vi "OD.vi"() -> ()   [LabVIEW 2012]
uses:
  <vilib>/Instr/_visa.llb/VISA Find Search Mode.ctl
  <vilib>/Utility/file.llb/Read From Spreadsheet File (string).vi
  <vilib>/Utility/file.llb/Write To Spreadsheet File (string).vi
  <vilib>/Utility/file.llb/Write To Spreadsheet File (DBL).vi
  <userlib>/SPECcon/SPECcon.lvlib
panel:
  out "Dark 2":dbl[](array[numeric])
  in  "DarkBefore":bool
  in  "Interval in minutes":dbl
  out "Absorbance [AU] vs. Wavelength [nm]":cluster{dbl[], dbl[]}[](graph)
  in  "Reset the graph for\nnext run":bool
  out "Dark":dbl[](array[numeric])
  out "Reference":dbl[](array[numeric])
  out "Connected?":bool
  out "Identified?":bool
  in  "to":i32=1050
  in  "from":i32=350
  in  "Run Python Script\non 'log_OD.txt'":bool
  in  "Automatic\nMeasurement":bool
  out "Samples Raw Data":dbl[][][](array[numeric])
  out "Command sent":string
  out "Raw Data":string
  in  "Average":i32=10
  in  "Integration Time":i32=100
  out "Number of bytes read":i32
  out "info out":string
  out "info return":i32
  in  "Connect to this port?":bool caption="Connect to this port"
  in  "index":i32
  out "Port":string caption="element"
  out "firmware out":string
  # "Connection"
  # "Data Acquisition"
  # "Measurement Settings"
  # "Wavelength Range (nm)"
  # "-"
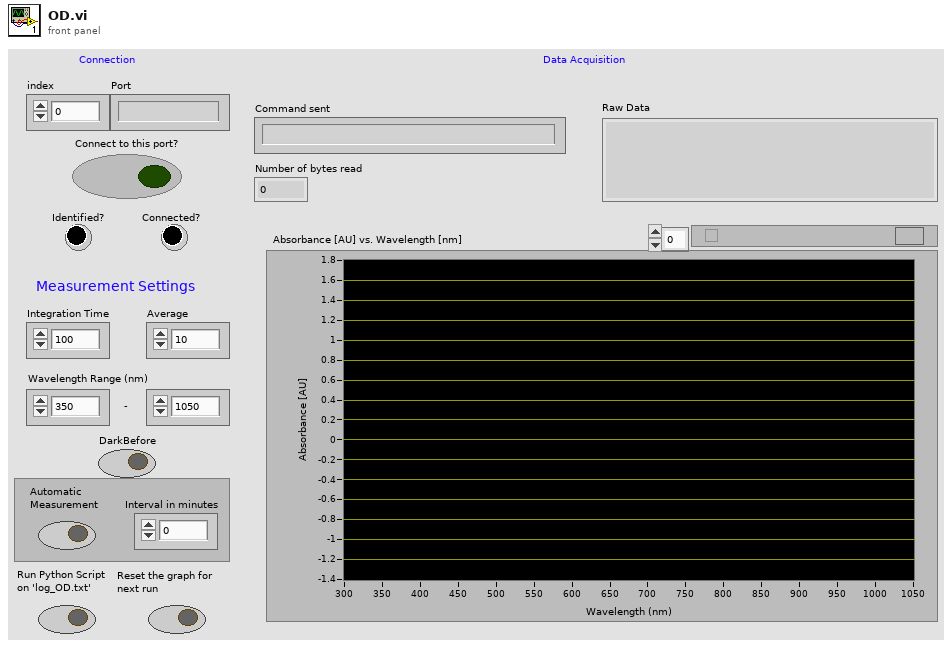
[diagram p1: front panel]
types:
  T1 = typedef "VISA Find Search Mode.ctl" = u32
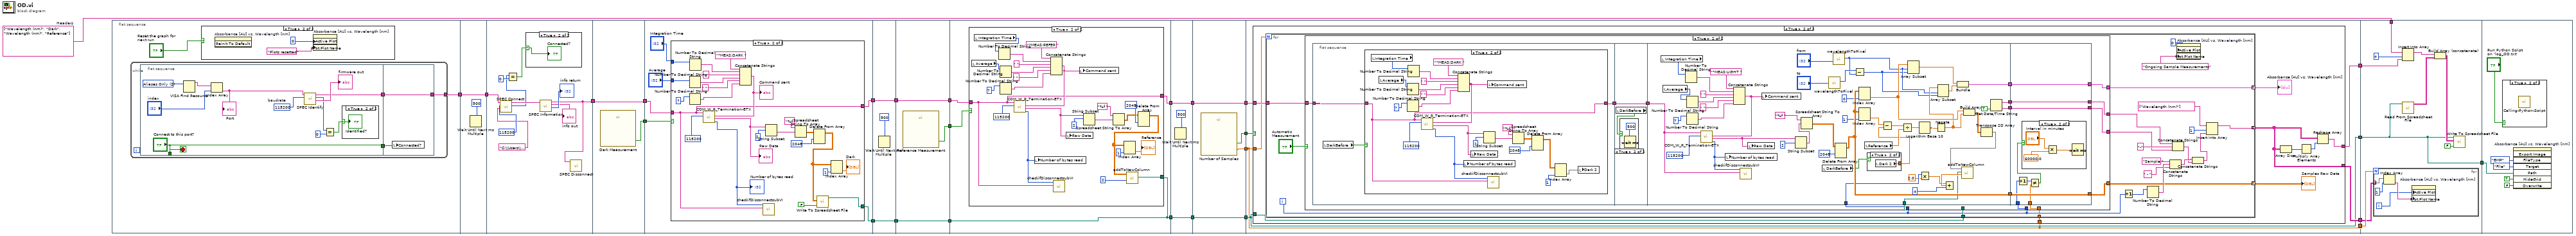
[diagram p0: block diagram]
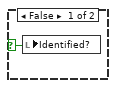
[diagram p3: hidden frame]
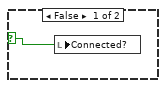
[diagram p4: hidden frame]
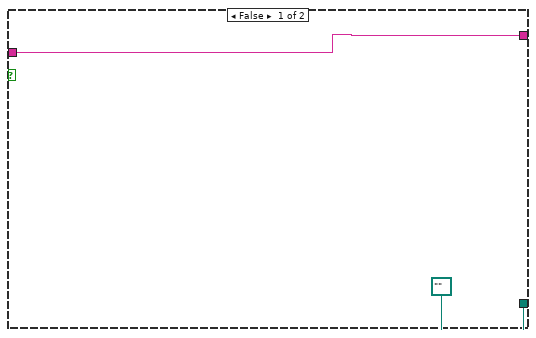
[diagram p5: hidden frame]
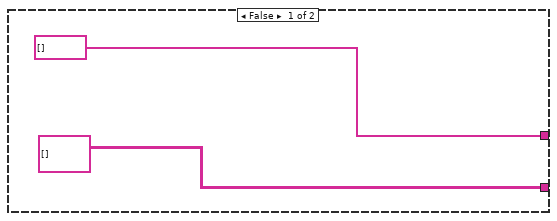
[diagram p7: hidden frame]
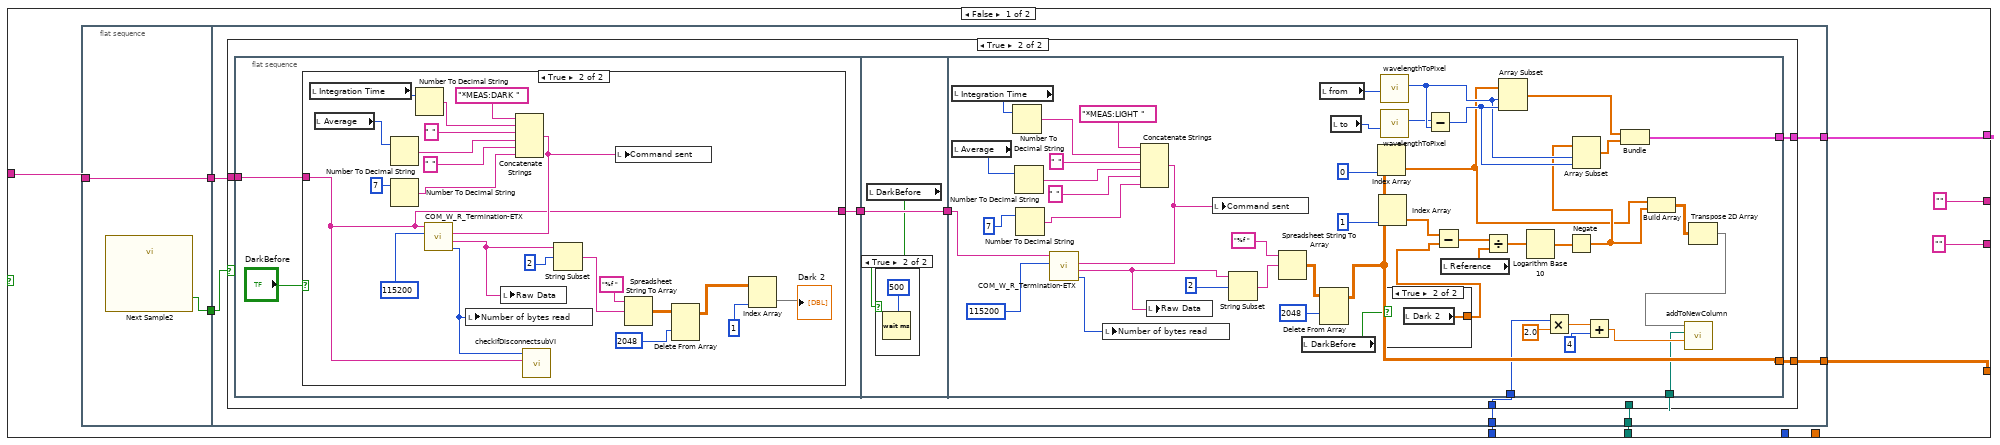
[diagram p8: hidden frame]
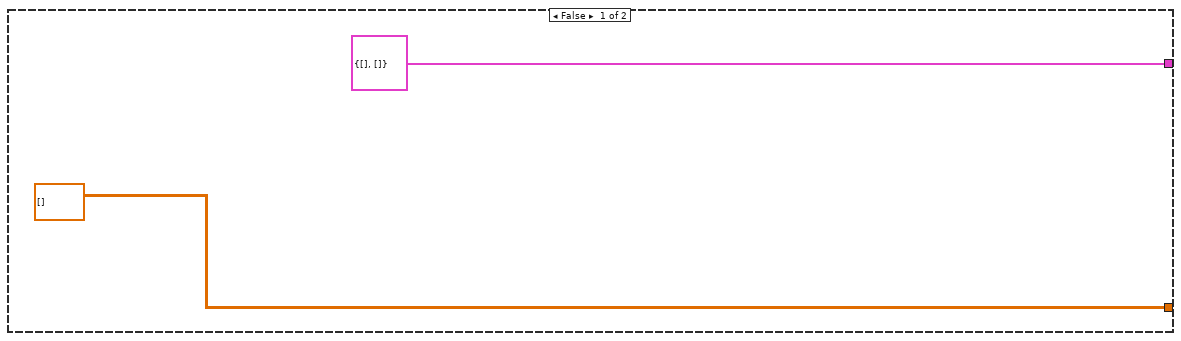
[diagram p9: hidden frame]
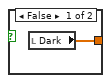
[diagram p12: hidden frame]
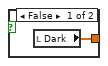
[diagram p15: hidden frame]
diagram:
  w5 = string[] ["Wavelength (nm)", "Dark", "Wavelength (nm)", "Reference"]  # Headers
  n1 = flat-sequence {
    tunnel: [w28] -> w26
    tunnel: w26 -> [w50]
    tunnel: [w50] -> w25
    tunnel: w25 -> [w58]
    tunnel: [w55] -> w16
    tunnel: [w65] -> w24
    tunnel: w16 -> [w65]
    tunnel: [w64] -> w15
    tunnel: w24 -> [w70]
    tunnel: w15 -> [w71]
    tunnel: [w67] -> w13
    tunnel: [w66] -> w7
    tunnel: [w99] -> w22
    tunnel: w13 -> [w99]
    tunnel: [w98] -> w8
    tunnel: w7 -> [w98]
    tunnel: [w103] -> w23
    tunnel: w22 -> [w103]
    tunnel: [w102] -> w21
    tunnel: [w101] -> w9
    tunnel: w8 -> [w101]
    tunnel: w23 -> [w107]
    tunnel: w21 -> [w106]
    tunnel: [w105] -> w14
    tunnel: [w104] -> w10
    tunnel: w9 -> [w104]
    tunnel: [w134] -> w17
    tunnel: w14 -> [w134]
    tunnel: [w133] -> w11
    tunnel: w10 -> [w133]
    tunnel: [w139] -> w20
    tunnel: [w138] -> w19
    tunnel: [w137] -> w18
    tunnel: w17 -> [w137]
    tunnel: [w136] -> w12
    tunnel: w11 -> [w136]
    tunnel: w20 -> [w145]
    tunnel: w19 -> [w140]
    tunnel: w18 -> [w144]
    tunnel: w12 -> [w141]
    tunnel: [w143] -> w6
    tunnel: [w140] -> w4
    tunnel: [w142] -> w3
    tunnel: [w141] -> w1
    tunnel: w5 -> [w400]
    tunnel: w6 -> [w398]
    tunnel: w4 -> [w393]
    tunnel: w3 -> [w392]
    tunnel: [w391] -> w2
    tunnel: w1 -> [w391]
    tunnel: w2 -> [w405]
    frame #0 {
      n2 = while {
        tunnel: [w34] -> w28
        stop <- w33 stop-if-true
        n3 = flat-sequence {
          tunnel: ["Connect to this port?"] -> w33
          tunnel: [w40] -> w32
          tunnel: ["Connect to this port?"] -> w31
          tunnel: [w49] -> w34
          tunnel: w32 -> [w49]
          tunnel: w31 -> [w48]
          frame #0 {
            w42 = T1 2 items=["Canonical Names Only"=0, "Aliases Only"=2, "Include Matching Aliases"=3, "Include All Aliases"=4] ("Search Mode")
            w45 = 115200  # baudrate
            n4 = VISA Find Resource(10:w42) -> (3:w41:string[])  [unwired: 2 in, 2 out]
            n5 = Index Array(array=w41, index="index") -> (element=w39:string)
            "Port" <- w39
            n6 = call <userlib>:"SPEC Identify.vi"("baudrate_or_mode"=w45, "port_number"=w39) -> ("firmware out"=→"firmware out":string, "function return"=w38:i32, "port_number out"=w40:string)  [unwired: 7 in]
            n7 = Equal?(x=w38, y=0) -> (x = y?=w36:bool)
            n8 = case shown="True" w36 {
              selector: w36 -> [w46 w47]
              frame False {
                n9 = local write "Identified?"(w46) -> ()
              }
              frame True {
                "Identified?" <- w47
              }
            }
          }
          frame #1 {
            n10 = local write "Connected?"(w48) -> ()
          }
        }
      }
      n11 = case shown="True" "Reset the graph for\nnext run" {
        frame False {
        }
        frame True {
          n12 = invoke on="Absorbance [AU] vs. Wavelength [nm]" class="XYGraph (strict)" method="Reinit To Default"() -> ()  [unwired: 3 in, 3 out]
          n13 = property on="Absorbance [AU] vs. Wavelength [nm]" class="XYGraph (strict)"("Active Plot"=u32 0, "Plot.Plot Name"="Plots resetted") -> ()  [unwired: 2 in, 2 out]
        }
      }
    }
    frame #1 {
      n14 = Wait Until Next ms Multiple(millisecond multiple=u32 500) -> ()  [unwired: 1 out]
    }
    frame #2 {
      n15 = call <userlib>:"SPEC Connect.vi"("filename"="C:\\Users\\Frederic Schmitt\\Desktop\\GE\\Optical Density - Sinan\\SPECview\\SPECcon_1.3\\example_CS.txt", "baudrate"=115200, "port_number"=w58) -> ("function return"=w52:i32, "port_number out"=w59:string)  [unwired: 6 in, 1 out]
      n16 = Equal?(x=w52, y=0) -> (x = y?=w53:bool)
      n17 = case shown="True" w53 {
        selector: w53 -> [w62 w63]
        frame False {
          n18 = local write "Connected?"(w62) -> ()
        }
        frame True {
          "Connected?" <- w63
        }
      }
      n19 = call <userlib>:"SPEC Information.vi"("port_number"=w59) -> ("function return"=→"info return":i32, "info out"=→"info out":string, "port_number out"=w55:string)  [unwired: 8 in]
      n20 = call <userlib>:"SPEC Disconnect.vi"("port_number"=w55) -> ()  [unwired: 9 in, 2 out]
    }
    frame #3 {
      n21 = call "Dark Measurement"() -> ("Sure"=w64:bool)  [unwired: 18 in, 1 out]
    }
    frame #4 {
      n22 = case shown="True" w71 {
        tunnel: w70 -> [w73 w75]
        tunnel: [w73 w75] -> w67
        tunnel: "Integration Time" -> [_ w89]
        tunnel: "Average" -> [_ w88]
        tunnel: [path "" ("new file path (Not A Path if cancelled)") w74] -> w66
        frame False {
        }
        frame True {
          n23 = Number To Decimal String(number=w88) -> (decimal integer string=w93:string)  [unwired: 1 in]
          n24 = Number To Decimal String(number=7) -> (decimal integer string=w91:string)  [unwired: 1 in]
          n25 = Number To Decimal String(number=w89) -> (decimal integer string=w95:string)  [unwired: 1 in]
          n26 = Concatenate Strings("*MEAS:DARK ", w95, " ", w93, " ", w91) -> (w80:string)
          "Command sent" <- w80
          n27 = call "COM_W_R_Termination-ETX.vi"("VISA resource name"=w75, "baud rate"=u32 115200, "string to write"=w80) -> ("read string"=w86:string, "return count"=w79:u32)  [unwired: 6 in]
          "Number of bytes read" <- w79
          "Raw Data" <- w86
          n28 = call "checkifDisconnectsubVI.vi"("port_number in"=w75, "function return 3"=w79) -> ()  [unwired: 10 in]
          n29 = String Subset(string=w86, offset (0)=2 ("offset")) -> (substring=w84:string)  [unwired: 1 in]
          n30 = Spreadsheet String To Array(format string="%f ", spreadsheet string=w84) -> (array=w81:dbl[][])  [unwired: 2 in]
          n31 = Delete From Array(array=w81, index (row)=2048) -> (array with subset deleted=w77:dbl[][])  [unwired: 2 in, 1 out]
          n32 = call-poly <vilib>:"Write To Spreadsheet File.vi"("append to file? (new file:F)"=FALSE, "2D data"=w77) -> ("new file path (Not A Path if cancelled)"=w74:path)  [unwired: 6 in]
          n33 = Index Array(array=w77, index (col)=1 ("disabled index (col)")) -> (element=→"Dark":dbl[])  [unwired: 1 in]
        }
      }
    }
    frame #5 {
      n34 = Wait Until Next ms Multiple(millisecond multiple=u32 500) -> ()  [unwired: 1 out]
    }
    frame #6 {
      n35 = call "Reference Measurement"() -> ("Sure"=w102:bool)  [unwired: 18 in, 1 out]
    }
    frame #7 {
      n36 = case shown="True" w106 {
        tunnel: w107 -> [w108 w110]
        tunnel: [w108 w110] -> w105
        tunnel: w104 -> [_ w109]
        frame False {
        }
        frame True {
          n37 = local read "Average"() -> (w124:i32)
          n38 = local read "Integration Time"() -> (w123:i32)
          n39 = Number To Decimal String(number=w123) -> (decimal integer string=w130:string)  [unwired: 1 in]
          n40 = Number To Decimal String(number=w124) -> (decimal integer string=w128:string)  [unwired: 1 in]
          n41 = Number To Decimal String(number=7) -> (decimal integer string=w126:string)  [unwired: 1 in]
          n42 = Concatenate Strings("*MEAS:REFER ", w130, " ", w128, " ", w126) -> (w116:string)
          n43 = call "COM_W_R_Termination-ETX.vi"("VISA resource name"=w110, "baud rate"=u32 115200, "string to write"=w116) -> ("read string"=w115:string, "return count"=w114:u32)  [unwired: 6 in]
          n44 = local write "Number of bytes read"(w114) -> ()
          n45 = call "checkifDisconnectsubVI.vi"("port_number in"=w110, "function return 3"=w114) -> ()  [unwired: 10 in]
          n46 = local write "Raw Data"(w115) -> ()
          n47 = local write "Command sent"(w116) -> ()
          n48 = String Subset(string=w115, offset (0)=2 ("offset")) -> (substring=w120:string)  [unwired: 1 in]
          n49 = Spreadsheet String To Array(format string="%f ", spreadsheet string=w120) -> (array=w117:dbl[][])  [unwired: 2 in]
          n50 = Delete From Array(array=w117, index (row)=2048) -> (array with subset deleted=w113:dbl[][])  [unwired: 2 in, 1 out]
          n51 = Index Array(array=w113, index (col)=1 ("disabled index (col)")) -> (element=→"Reference":dbl[])  [unwired: 1 in]
          n52 = call "addToNewColumn.vi"("disabled index (col)"=2, "new file path (Not A Path if cancelled)"=w109, "Array"=w113) -> ()  [unwired: 9 in]
        }
      }
    }
    frame #8 {
      n53 = Wait Until Next ms Multiple(millisecond multiple=u32 500) -> ()  [unwired: 1 out]
    }
    frame #9 {
      n54 = call "Number of Samples"() -> ("number_samples"=w138:dbl, "OK"=w139:bool)  [unwired: 17 in, 1 out]
    }
    frame #10 {
      n55 = case shown="True" w145 {
        tunnel: w140 -> [_ w155]
        tunnel: w144 -> [_ w157]
        tunnel: w141 -> [_ w148]
        tunnel: [string[] [] w153] -> w143
        tunnel: [string[][] [] ("array") w150] -> w142
        tunnel: w140 -> [_ w149]
        frame False {
        }
        frame True {
          n56 = for {
            N: w155 -> [_]
            tunnel: w157 -> [w179]
            tunnel: [w160] -> w156 mode=indexing
            tunnel: w148 -> [w178]
            tunnel: [w173] -> w150 mode=indexing
            tunnel: [w167] -> w151 mode=indexing
            tunnel: w149 -> [w158]
            i -> [w159]
            n57 = case shown="True" "Automatic\nMeasurement" {
              tunnel: w179 -> [w186 w298]
              tunnel: [w185 w284] -> w160
              tunnel: w178 -> [w183 w297]
              tunnel: w159 -> [w184 w296]
              tunnel: [w182 w285] -> w167
              tunnel: ["" ("date string") w286] -> w162
              tunnel: ["" ("time string") w287] -> w161
              tunnel: w159 -> [_ w289]
              tunnel: w158 -> [_ w288]
              frame False {
                n58 = flat-sequence {
                  tunnel: w186 -> [w190]
                  tunnel: [w190] -> w188
                  tunnel: [w189] -> w187
                  tunnel: w188 -> [w196]
                  tunnel: w187 -> [w195]
                  tunnel: [w194] -> w185
                  tunnel: w184 -> [w191]
                  tunnel: w183 -> [w193]
                  tunnel: [w192] -> w182
                  frame #0 {
                    n59 = call "Next Sample2"() -> ("OK"=w189:bool)  [unwired: 18 in, 1 out]
                  }
                  frame #1 {
                    n60 = case shown="True" w195 {
                      tunnel: w196 -> [_ w204]
                      tunnel: [dbl[][] [] w205] -> w194
                      tunnel: w191 -> [_ w199]
                      tunnel: w193 -> [_ w200]
                      tunnel: [cluster{dbl[], dbl[]} {[], []} w201] -> w192
                      frame False {
                      }
                      frame True {
                        n61 = flat-sequence {
                          tunnel: w204 -> [w207]
                          tunnel: [w206] -> w203
                          tunnel: w203 -> [w233]
                          tunnel: [w233] -> w202
                          tunnel: [w242] -> w205
                          tunnel: w199 -> [w235]
                          tunnel: w200 -> [w241]
                          tunnel: w202 -> [w240]
                          tunnel: [w239] -> w201
                          frame #0 {
                            n62 = case shown="True" "DarkBefore" {
                              tunnel: w207 -> [w209 w211]
                              tunnel: [w209 w211] -> w206
                              frame False {
                              }
                              frame True {
                                n63 = local read "Integration Time"() -> (w216:i32)
                                n64 = local read "Average"() -> (w215:i32)
                                n65 = Number To Decimal String(number=w215) -> (decimal integer string=w228:string)  [unwired: 1 in]
                                n66 = Number To Decimal String(number=7) -> (decimal integer string=w226:string)  [unwired: 1 in]
                                n67 = Number To Decimal String(number=w216) -> (decimal integer string=w230:string)  [unwired: 1 in]
                                n68 = Concatenate Strings("*MEAS:DARK ", w230, " ", w228, " ", w226) -> (w214:string)
                                n69 = call "COM_W_R_Termination-ETX.vi"("VISA resource name"=w211, "baud rate"=u32 115200, "string to write"=w214) -> ("read string"=w212:string, "return count"=w213:u32)  [unwired: 6 in]
                                n70 = local write "Number of bytes read"(w213) -> ()
                                n71 = local write "Raw Data"(w212) -> ()
                                n72 = call "checkifDisconnectsubVI.vi"("port_number in"=w211, "function return 3"=w213) -> ()  [unwired: 10 in]
                                n73 = String Subset(string=w212, offset (0)=2 ("offset")) -> (substring=w221:string)  [unwired: 1 in]
                                n74 = local write "Command sent"(w214) -> ()
                                n75 = Spreadsheet String To Array(format string="%f ", spreadsheet string=w221) -> (array=w220:dbl[][])  [unwired: 2 in]
                                n76 = Delete From Array(array=w220, index (row)=2048) -> (array with subset deleted=w218:dbl[][])  [unwired: 2 in, 1 out]
                                n77 = Index Array(array=w218, index (col)=1 ("disabled index (col)")) -> (element=→"Dark 2":dbl[])  [unwired: 1 in]
                              }
                            }
                          }
                          frame #1 {
                            n78 = local read "DarkBefore"() -> (w232:bool)
                            n79 = case shown="True" w232 {
                              frame False {
                              }
                              frame True {
                                n80 = Wait (ms)(milliseconds to wait=u32 500) -> ()  [unwired: 1 out]
                              }
                            }
                          }
                          frame #2 {
                            n81 = local read "Integration Time"() -> (w273:i32)
                            n82 = local read "Average"() -> (w272:i32)
                            n83 = Number To Decimal String(number=w273) -> (decimal integer string=w245:string)  [unwired: 1 in]
                            n84 = Number To Decimal String(number=w272) -> (decimal integer string=w247:string)  [unwired: 1 in]
                            n85 = Number To Decimal String(number=7) -> (decimal integer string=w249:string)  [unwired: 1 in]
                            n86 = Concatenate Strings("*MEAS:LIGHT ", w245, " ", w247, " ", w249) -> (w274:string)
                            n87 = call "COM_W_R_Termination-ETX.vi"("VISA resource name"=w240, "baud rate"=u32 115200, "string to write"=w274) -> ("read string"=w236:string, "return count"=w275:u32)  [unwired: 6 in]
                            n88 = local write "Number of bytes read"(w275) -> ()
                            n89 = local write "Raw Data"(w236) -> ()
                            n90 = local write "Command sent"(w274) -> ()
                            n91 = String Subset(string=w236, offset (0)=2 ("offset")) -> (substring=w253:string)  [unwired: 1 in]
                            n92 = Spreadsheet String To Array(format string="%f ", spreadsheet string=w253) -> (array=w270:dbl[][])  [unwired: 2 in]
                            n93 = local read "DarkBefore"() -> (w238:bool)
                            n94 = local read "from"() -> (w277:i32)
                            n95 = Delete From Array(array=w270, index (row)=2048) -> (array with subset deleted=w242:dbl[][])  [unwired: 2 in, 1 out]
                            n96 = local read "to"() -> (w278:i32)
                            n97 = Index Array(array=w242, index (col)=0 ("disabled index (col)")) -> (element=w266:dbl[])  [unwired: 1 in]
                            n98 = Index Array(array=w242, index (col)=1 ("disabled index (col)")) -> (element=w255:dbl[])  [unwired: 1 in]
                            n99 = call "wavelengthToPixel.vi"("w"=w277) -> ("r1"=w280:i32)  [unwired: 8 in, 1 out]
                            n100 = call "wavelengthToPixel.vi"("w"=w278) -> ("r1"=w279:i32)  [unwired: 8 in, 1 out]
                            n101 = case shown="True" w238 {
                              tunnel: [w282 w283] -> w237
                              frame False {
                                n102 = local read "Dark"() -> (w282:dbl[])
                              }
                              frame True {
                                n103 = local read "Dark 2"() -> (w283:dbl[])
                              }
                            }
                            n104 = Subtract(x=w279, y=w280) -> (x-y=w281:i32)
                            n105 = Subtract(x=w255, y=w237) -> (x-y=w256:dbl[])
                            n106 = local read "Reference"() -> (w276:dbl[])
                            n107 = Divide(x=w256, y=w276) -> (x/y=w257:dbl[])
                            n108 = Array Subset(array=w266, index=w280, length=w281) -> (w267:dbl[])
                            n109 = Logarithm Base 10(1:w257) -> (0:w258:dbl[])
                            n110 = Multiply(x=w235, y=2.0) -> (x*y=w265:dbl)
                            n111 = Negate(x=w258) -> (-x=w268:dbl[])
                            n112 = Array Subset(array=w268, index=w280, length=w281) -> (w269:dbl[])
                            n113 = Add(x=w265, y=4) -> (x+y=w261:dbl)
                            n114 = Bundle(w267, w269) -> (w239:cluster{dbl[], dbl[]})  [unwired: 1 in]
                            n115 = Build Array(w266, w268) -> (w262:dbl[][])
                            n116 = Transpose 2D Array(2D array=w262) -> (transposed array=w263:dbl[][])
                            n117 = call "addToNewColumn.vi"("disabled index (col)"=w261, "new file path (Not A Path if cancelled)"=w241, "Array"=w263) -> ()  [unwired: 9 in]
                          }
                        }
                      }
                    }
                  }
                }
              }
              frame True {
                n118 = flat-sequence {
                  tunnel: w298 -> [w301]
                  tunnel: [w300] -> w294
                  tunnel: [w326] -> w295
                  tunnel: w294 -> [w326]
                  tunnel: w297 -> [w332]
                  tunnel: w296 -> [w376]
                  tunnel: w295 -> [w330]
                  tunnel: [w377] -> w293
                  tunnel: [w345] -> w292
                  tunnel: [w336] -> w291
                  tunnel: [w335] -> w290
                  tunnel: [w384] -> w287
                  tunnel: [w385] -> w286
                  tunnel: [w386] -> w285
                  tunnel: [w387] -> w284
                  tunnel: w293 -> [w387]
                  tunnel: w292 -> [w386]
                  tunnel: w291 -> [w385]
                  tunnel: w290 -> [w384]
                  tunnel: w289 -> [w382]
                  tunnel: w288 -> [w381]
                  frame #0 {
                    n119 = local read "DarkBefore"() -> (w299:bool)
                    n120 = case shown="True" w299 {
                      tunnel: w301 -> [w302 w303]
                      tunnel: [w302 w303] -> w300
                      frame False {
                      }
                      frame True {
                        n121 = local read "Integration Time"() -> (w307:i32)
                        n122 = local read "Average"() -> (w306:i32)
                        n123 = Number To Decimal String(number=w306) -> (decimal integer string=w320:string)  [unwired: 1 in]
                        n124 = Number To Decimal String(number=7) -> (decimal integer string=w318:string)  [unwired: 1 in]
                        n125 = Number To Decimal String(number=w307) -> (decimal integer string=w322:string)  [unwired: 1 in]
                        n126 = Concatenate Strings("*MEAS:DARK ", w322, " ", w320, " ", w318) -> (w309:string)
                        n127 = call "COM_W_R_Termination-ETX.vi"("VISA resource name"=w303, "baud rate"=u32 115200, "string to write"=w309) -> ("read string"=w305:string, "return count"=w308:u32)  [unwired: 6 in]
                        n128 = local write "Number of bytes read"(w308) -> ()
                        n129 = local write "Raw Data"(w305) -> ()
                        n130 = String Subset(string=w305, offset (0)=2 ("offset")) -> (substring=w314:string)  [unwired: 1 in]
                        n131 = call "checkifDisconnectsubVI.vi"("port_number in"=w303, "function return 3"=w308) -> ()  [unwired: 10 in]
                        n132 = local write "Command sent"(w309) -> ()
                        n133 = Spreadsheet String To Array(format string="%f ", spreadsheet string=w314) -> (array=w312:dbl[][])  [unwired: 2 in]
                        n134 = Delete From Array(array=w312, index (row)=2048) -> (array with subset deleted=w310:dbl[][])  [unwired: 2 in, 1 out]
                        n135 = Index Array(array=w310, index (col)=1 ("disabled index (col)")) -> (element=w304:dbl[])  [unwired: 1 in]
                        n136 = local write "Dark 2"(w304) -> ()
                      }
                    }
                  }
                  frame #1 {
                    n137 = local read "DarkBefore"() -> (w325:bool)
                    n138 = case shown="True" w325 {
                      frame False {
                      }
                      frame True {
                        n139 = Wait (ms)(milliseconds to wait=u32 500) -> ()  [unwired: 1 out]
                      }
                    }
                  }
                  frame #2 {
                    n140 = local read "Integration Time"() -> (w367:i32)
                    n141 = local read "Average"() -> (w366:i32)
                    n142 = Number To Decimal String(number=w367) -> (decimal integer string=w373:string)  [unwired: 1 in]
                    n143 = Number To Decimal String(number=w366) -> (decimal integer string=w371:string)  [unwired: 1 in]
                    n144 = Number To Decimal String(number=7) -> (decimal integer string=w369:string)  [unwired: 1 in]
                    n145 = Concatenate Strings("*MEAS:LIGHT ", w373, " ", w371, " ", w369) -> (w339:string)
                    n146 = call "COM_W_R_Termination-ETX.vi"("VISA resource name"=w330, "baud rate"=u32 115200, "string to write"=w339) -> ("read string"=w329:string, "return count"=w331:u32)  [unwired: 6 in]
                    n147 = local write "Number of bytes read"(w331) -> ()
                    n148 = call "checkifDisconnectsubVI.vi"("port_number in"=w330, "function return 3"=w331) -> ()  [unwired: 10 in]
                    n149 = local write "Raw Data"(w329) -> ()
                    n150 = local write "Command sent"(w339) -> ()
                    n151 = String Subset(string=w329, offset (0)=2 ("offset")) -> (substring=w328:string)  [unwired: 1 in]
                    n152 = Spreadsheet String To Array(format string="%f ", spreadsheet string=w328) -> (array=w347:dbl[][])  [unwired: 2 in]
                    n153 = local read "DarkBefore"() -> (w334:bool)
                    n154 = call "wavelengthToPixel.vi"("w"="to") -> ("r1"=w342:i32)  [unwired: 8 in, 1 out]
                    n155 = call "wavelengthToPixel.vi"("w"="from") -> ("r1"=w341:i32)  [unwired: 8 in, 1 out]
                    n156 = Delete From Array(array=w347, index (row)=2048) -> (array with subset deleted=w377:dbl[][])  [unwired: 2 in, 1 out]
                    n157 = Subtract(x=w342, y=w341) -> (x-y=w340:i32)
                    n158 = Index Array(array=w377, index (col)=0 ("disabled index (col)")) -> (element=w351:dbl[])  [unwired: 1 in]
                    n159 = Index Array(array=w377, index (col)=1 ("disabled index (col)")) -> (element=w362:dbl[])  [unwired: 1 in]
                    n160 = local read "Reference"() -> (w338:dbl[])
                    n161 = case shown="True" w334 {
                      tunnel: [w378 w379] -> w333
                      frame False {
                        n162 = local read "Dark"() -> (w378:dbl[])
                      }
                      frame True {
                        n163 = local read "Dark 2"() -> (w379:dbl[])
                      }
                    }
                    n164 = Subtract(x=w362, y=w333) -> (x-y=w361:dbl[])
                    n165 = Divide(x=w361, y=w338) -> (x/y=w360:dbl[])
                    n166 = Array Subset(array=w351, index=w341, length=w340) -> (w350:dbl[])
                    n167 = Logarithm Base 10(1:w360) -> (0:w359:dbl[])
                    n168 = Multiply(x=w376, y=2.0) -> (x*y=w352:dbl)
                    n169 = Negate(x=w359) -> (-x=w349:dbl[])
                    n170 = Array Subset(array=w349, index=w341, length=w340) -> (w348:dbl[])
                    n171 = Add(x=w352, y=4) -> (x+y=w356:dbl)
                    n172 = Bundle(w350, w348) -> (w345:cluster{dbl[], dbl[]})  [unwired: 1 in]
                    n173 = Build Array(w351, w349) -> (w355:dbl[][])
                    n174 = Transpose 2D Array(2D array=w355) -> (transposed array=w354:dbl[][])
                    n175 = call "addToNewColumn.vi"("disabled index (col)"=w356, "new file path (Not A Path if cancelled)"=w332, "Array"=w354) -> ()  [unwired: 9 in]
                    n176 = Get Date/Time String(want seconds? (F)=TRUE) -> (date string=w336:string, time string=w335:string)  [unwired: 2 in]
                  }
                  frame #3 {
                    n177 = Increment(x=w382) -> (x+1=w383:i32)
                    n178 = Not Equal?(x=w383, y=w381) -> (x != y?=w380:bool)
                    n179 = case shown="True" w380 {
                      frame False {
                      }
                      frame True {
                        n180 = Multiply(x="Interval in minutes", y=60000.0 ("x")) -> (x*y=w390:dbl)
                        n181 = Wait (ms)(milliseconds to wait=w390) -> ()  [unwired: 1 out]
                      }
                    }
                  }
                }
              }
            }
            n182 = Increment(x=w159) -> (x+1=w166:i32)
            n183 = Number To Decimal String(number=w166) -> (decimal integer string=w172:string)  [unwired: 1 in]
            n184 = Concatenate Strings("Sample ", w172, " - " ("string")) -> (w169:string)
            n185 = Concatenate Strings(w162, "-" ("string"), w161) -> (w168:string)
            n186 = property on="Absorbance [AU] vs. Wavelength [nm]" class="XYGraph (strict)"("Active Plot"=u32 0, "Plot.Plot Name"="Ongoing Sample Measurements") -> ()  [unwired: 2 in, 2 out]
            n187 = Concatenate Strings(w169, w168) -> (w165:string)
            n188 = Insert Into Array(array=string[] ["Wavelength (nm)"], index=1, new element=w165) -> (w173:string[])
          }
          "Samples Raw Data" <- w156
          "Absorbance [AU] vs. Wavelength [nm]" <- w151
          n189 = Array Size(array=w150) -> (size(s)=w152:i32[])
          n190 = Multiply Array Elements(1:w152) -> (0:w154:i32)
          n191 = Reshape Array(w150, w154) -> (w153:string[])
        }
      }
    }
    frame #11 {
      n192 = for {
        N: w393 -> [_]
        tunnel: w392 -> [w404] mode=indexing
        i -> [w401]
        n193 = Index Array(array=w404, index=1) -> (element=w402:string)
        n194 = property on="Absorbance [AU] vs. Wavelength [nm]" class="XYGraph (strict)"("Active Plot"=w401, "Plot.Plot Name"=w402) -> ()  [unwired: 2 in, 2 out]
      }
      n195 = Insert Into Array(array=w400, index=4, new element=w398) -> (w397:string[])
      n196 = call-poly <vilib>:"Read From Spreadsheet File.vi"("file path (dialog if empty)"=w391) -> ("all rows"=w396:string[][])  [unwired: 6 in, 4 out]
      n197 = Build Array (concatenate)(w397, w396) -> (w395:string[][])
      n198 = call-poly <vilib>:"Write To Spreadsheet File.vi"("append to file? (new file:F)"=FALSE, "2D data"=w395, "file path (dialog if empty)"=w391) -> ()  [unwired: 5 in, 1 out]
    }
    frame #12 {
      n199 = case shown="True" "Run Python Script\non 'log_OD.txt'" {
        frame False {
        }
        frame True {
          n200 = call "Calling-Python-Script.vi"() -> ()  [unwired: 1 in]
        }
      }
      n201 = invoke on="Absorbance [AU] vs. Wavelength [nm]" class="XYGraph (strict)" method="Export Image"("FileType"=enum32{"BMP", "EPS", "EMF", "PICT"}."BMP" ("File Type"), "Target"=enum32{"File", "Clipboard"}."File", "Path"=w405, "HideGrid"=TRUE ("Hide Grid"), "Overwrite"=FALSE ("Always Overwrite")) -> ()  [unwired: 3 in, 8 out]
    }
  }
